vi "Start.vi"(0 "reference in":refnum<class "Direction.lvclass">, 5 "error in (no error)":errorcluster) -> (14 "reference out":refnum<class "Direction.lvclass">, 19 "error out":errorcluster)   [LabVIEW 2013, in "Direction.lvclass"]
uses:
  Direction.lvclass
  Dec_class/Dec.lvclass
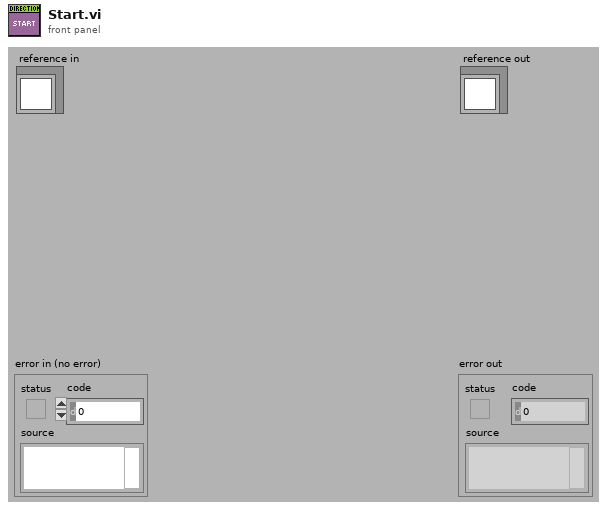
[diagram p1: front panel]
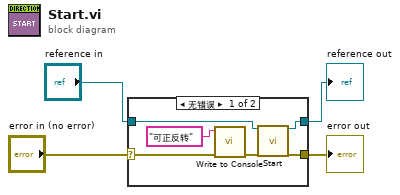
[diagram p0: block diagram]
diagram:
  n1 = case shown="无错误" "error in (no error)" {
    selector: "error in (no error)" -> [w7 w11]
    tunnel: [w9 w12] -> w2
    tunnel: "reference in" -> [w10 w12]
    tunnel: [w5 w11] -> w1
    frame No Error {
      n2 = call "Write to Console.vi"("error in (no error)"=w7, "Input"="可正反转") -> ("error out"=w6:errorcluster)  [unwired: 9 in]
      n3 = call-parent "Start.vi"("reference in"=w10, "error in (no error)"=w6) -> ("reference out"=w9:refnum<class "Direction.lvclass">, "error out"=w5:errorcluster)  [unwired: 16 in]
    }
    frame Error {
    }
  }
  "error out" <- w1
  "reference out" <- w2
